vi "RangeDataFilesNm.vi"(8 "error in (no error)":errorcluster, 9 "Range_String":string="All" caption="Range String (yymmdd)", 10 "noms des fichiers":string[](array[string]), 11 "DataPath":path) -> (0 "error out":errorcluster, 2 "HdrFilesNames":path[](array[path]), 3 "DataPathOut":path)   [LabVIEW 2010]
uses:
  <vilib>/Utility/miscctls.llb/LVDateTimeRec.ctl
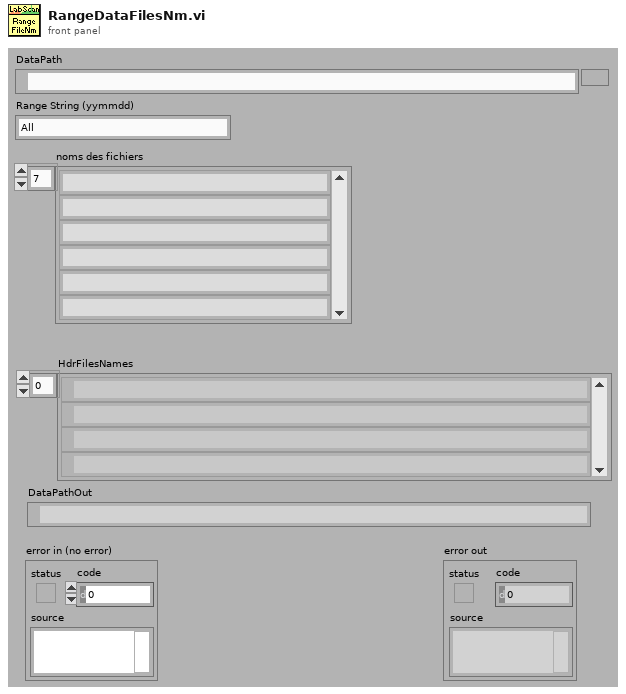
[diagram p1: front panel]
types:
  T1 = typedef "LVDateTimeRec.ctl" = cluster{"fractional second":dbl, "second":i32, "minute":i32, "hour":i32, "day of month":i32, "month":i32, "year":i32, "day of week":i32, "day of year":i32, "DST":i32}
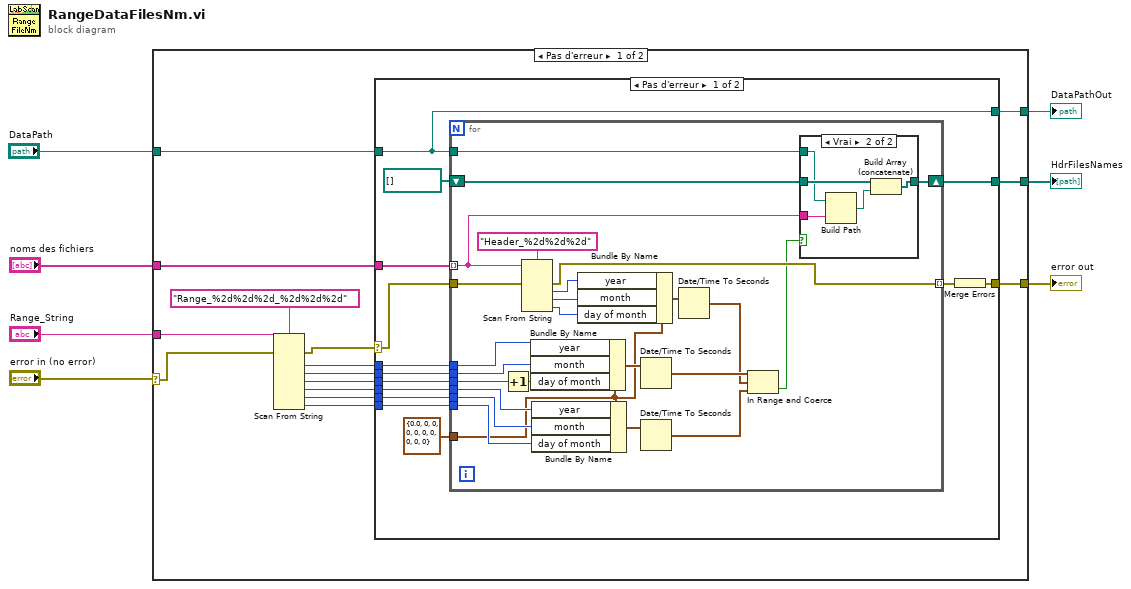
[diagram p0: block diagram]
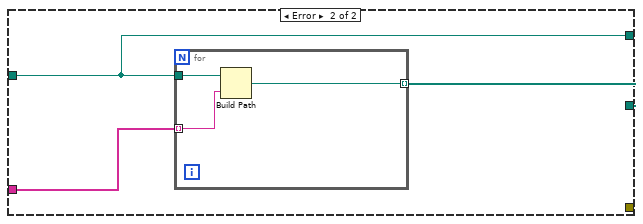
[diagram p3: hidden frame]
diagram:
  n1 = case shown="Pas d'erreur" "error in (no error)" {
    selector: "error in (no error)" -> [w11 w75]
    tunnel: "Range_String" -> [w22 _]
    tunnel: "noms des fichiers" -> [w21 _]
    tunnel: "DataPath" -> [w12 w74]
    tunnel: [w10 w75] -> w3
    tunnel: [w9 _] -> w2
    tunnel: [w8 w74] -> w1
    frame No Error {
      n2 = Scan From String(format string="Range_%2d%2d%2d_%2d%2d%2d" ("chaîne de format"), input string=w22, error in=w11) -> (error out=w13:errorcluster, output 1=w19:i32, output 2=w18:i32, output 3=w17:i32, output 4=w16:i32, output 5=w15:i32, output 6=w14:i32)  [unwired: 7 in, 2 out]
      n3 = case shown="Pas d'erreur" w13 {
        selector: w13 -> [w28 _]
        tunnel: w21 -> [w36 w70]
        tunnel: w19 -> [w35 _]
        tunnel: w18 -> [w34 _]
        tunnel: w17 -> [w33 _]
        tunnel: w16 -> [w32 _]
        tunnel: w15 -> [w31 _]
        tunnel: w14 -> [w30 _]
        tunnel: [w29 w69] -> w9
        tunnel: w12 -> [w24 w68]
        tunnel: [w26 _] -> w10
        tunnel: [w24 w68] -> w8
        frame No Error {
          n4 = for {
            tunnel: w36 -> [w58] mode=indexing
            tunnel: w35 -> [w55]
            tunnel: w34 -> [w53]
            tunnel: w33 -> [w54]
            tunnel: w32 -> [w51]
            tunnel: w31 -> [w50]
            tunnel: w30 -> [w49]
            shift-right: [w59] -> w29
            shift-left: path[] [] ("noms des fichiers") -> [w60]
            tunnel: w24 -> [w57]
            tunnel: w28 -> [w56]
            tunnel: [w44] -> w27 mode=indexing
            tunnel: T1 {"fractional second"=0.0, "second"=0, "minute"=0, "hour"=0, "day of month"=0, "month"=0, "year"=0, "day of week"=0, "day of year"=0, "DST"=0} ("cluster date/heure") -> [w43]
            n5 = Increment(x=w54) -> (x+1=w37:i32)
            n6 = Scan From String(format string="Header_%2d%2d%2d" ("chaîne de format"), input string=w58, error in=w56) -> (error out=w44:errorcluster, output 1=w47:i32, output 2=w46:i32, output 3=w45:i32)  [unwired: 4 in, 2 out]
            n7 = Bundle By Name(cluster=w43, "year"=w55, "month"=w53, "day of month"=w37) -> (w52:T1)
            n8 = Bundle By Name(cluster=w43, "year"=w51, "month"=w50, "day of month"=w49) -> (w48:T1)
            n9 = Bundle By Name(cluster=w43, "year"=w47, "month"=w46, "day of month"=w45) -> (w42:T1)
            n10 = Date/Time To Seconds(2:w52) -> (0:w41:timestamp)  [unwired: 1 in]
            n11 = Date/Time To Seconds(2:w48) -> (0:w39:timestamp)  [unwired: 1 in]
            n12 = Date/Time To Seconds(2:w42) -> (0:w40:timestamp)  [unwired: 1 in]
            n13 = In Range and Coerce(upper limit=w41, x=w40, lower limit=w39) -> (In Range?=w38:bool)  [unwired: 1 out]
            n14 = case shown="Vrai" w38 {
              tunnel: w60 -> [w62 w67]
              tunnel: [w62 w63] -> w59
              tunnel: w58 -> [_ w66]
              tunnel: w57 -> [_ w65]
              frame False {
              }
              frame True {
                n15 = Build Path(base path=w65, name or relative path=w66) -> (appended path=w64:path)
                n16 = Build Array (concatenate)(w67, w64) -> (w63:path[])
              }
            }
          }
          n17 = Merge Errors(w27) -> (w26:errorcluster)
        }
        frame Error {
          n18 = for {
            tunnel: w68 -> [w72]
            tunnel: w70 -> [w73] mode=indexing
            tunnel: [w71] -> w69 mode=indexing
            n19 = Build Path(base path=w72, name or relative path=w73) -> (appended path=w71:path)
          }
        }
      }
    }
    frame Error {
    }
  }
  "error out" <- w3
  "HdrFilesNames" <- w2
  "DataPathOut" <- w1
